vi "Compress Chirp.vi"(1 "Chirp":dbl[](array[numeric]), 2 "Array In":dbl[][](array[numeric])) -> (0 "Array Out":dbl[][](array[numeric]))   [LabVIEW 2022 SP3]
uses:
  <vilib>/Analysis/2dsp.llb/1D Convolution (DBL).vi
  <vilib>/Analysis/NI_AALPro.lvlib
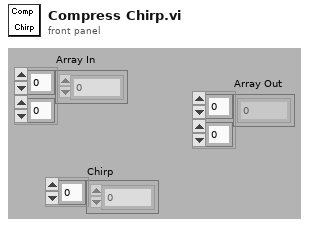
[diagram p1: front panel]
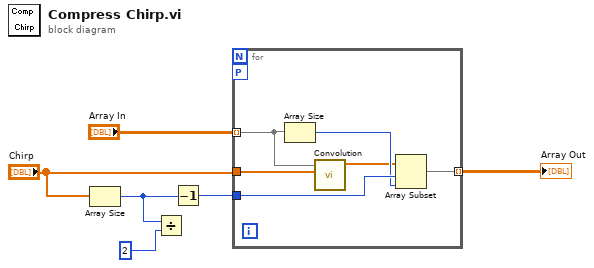
[diagram p0: block diagram]
diagram:
  n1 = Array Size(array="Chirp") -> (size(s)=w3:i32)
  n2 = Divide(x=w3, y=2) -> ()  [unwired: 1 out]
  n3 = Decrement(x=w3) -> (x-1=w2:i32)
  n4 = for {
    tunnel: "Array In" -> [w12] mode=indexing
    tunnel: [w11] -> w6 mode=indexing
    tunnel: "Chirp" -> [w10]
    tunnel: w2 -> [w9]
    workers-P: _ -> [_]
    n5 = Array Size(array=w12) -> (size(s)=w8:i32)
    n6 = call-poly <vilib>:"Convolution.vi"("Y"=w10, "X"=w12) -> ("X * Y"=w7:dbl[])  [unwired: 1 in, 8 out]
    n7 = Array Subset(array=w7, index=w9, length=w8) -> (w11:dbl[])
  }
  "Array Out" <- w6
